vi "SpectrumConfigDone.vi"(8 "error in (no error)":errorcluster, 11 "SpectrumAnalyzerUI in":refnum<class "SpectrumAnalyzerUI.lvclass">) -> (0 "error out":errorcluster, 3 "SpectrumAnalyzerUI out":refnum<class "SpectrumAnalyzerUI.lvclass">)   [LabVIEW 2023, in "SpectrumAnalyzerUI.lvlib" / "SpectrumAnalyzerUI.lvclass"]
uses:
  SpectrumAnalyzerUI.lvclass
  SpectrumAnalyzerUI.lvclass/SpectrumAnalyzerUI.ctl
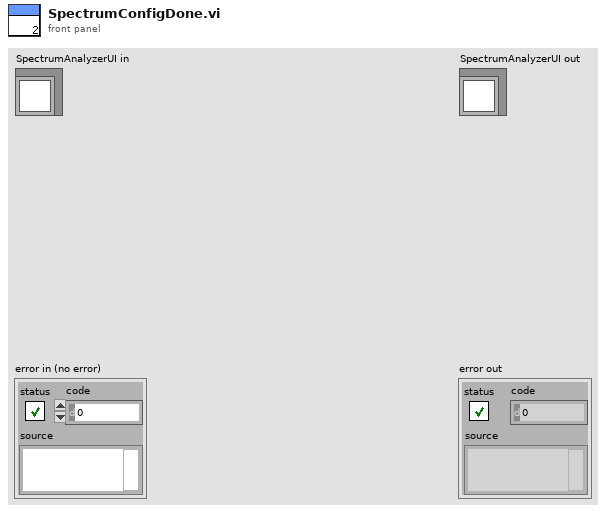
[diagram p1: front panel]
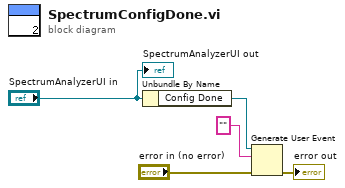
[diagram p0: block diagram]
diagram:
  n1 = Unbundle By Name("SpectrumAnalyzerUI in") -> ("Config Done"=w5:refnum<user-event>)
  n2 = Generate User Event(user event=w5, event data cluster="" ("event data"), error in="error in (no error)") -> (error out=→"error out":errorcluster)  [unwired: 1 in, 1 out]
  "SpectrumAnalyzerUI out" <- "SpectrumAnalyzerUI in"
